vi "get event specifications.vi"(8 "error in":errorcluster, 11 "module configuration in":refnum<class "TBM module configuration.lvclass">) -> (0 "error out":errorcluster, 2 "events":T1[](array[typedef]), 3 "module configuration out":refnum<class "TBM module configuration.lvclass">)   [LabVIEW 2013, in "TBM module configuration.lvclass"]
uses:
  TBM module configuration.lvclass
  event specification.ctl
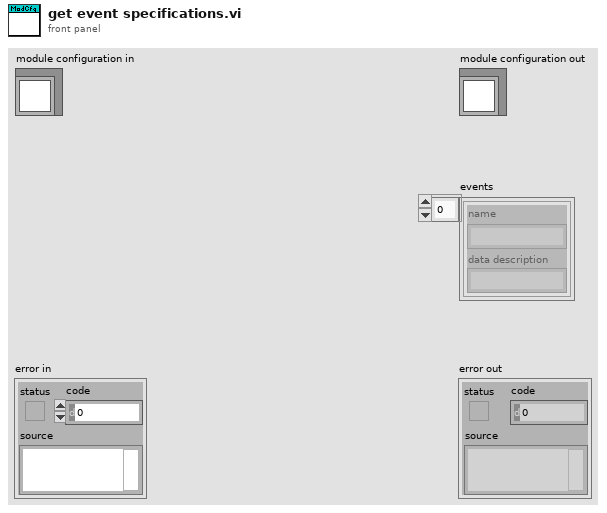
[diagram p1: front panel]
types:
  T1 = typedef "TBM module configuration.lvclass/event specification.ctl" = cluster{"name":string, "data description":string}
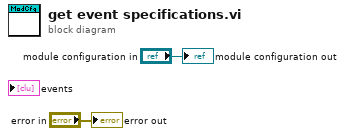
[diagram p0: block diagram]
diagram:
  "error out" <- "error in"
  "module configuration out" <- "module configuration in"
